vi "EDS test 02_2.vi"() -> ()   [LabVIEW 2020]
panel:
  out "max value":dbl
  in  "Ultrasonic 01":dbl
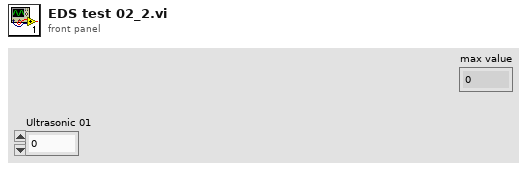
[diagram p1: front panel]
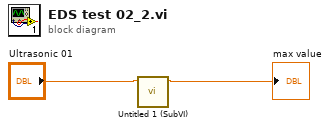
[diagram p0: block diagram]
diagram:
  n1 = call "Untitled 1 (SubVI).vi"("Ultrasonic 01"="Ultrasonic 01") -> ("Numeric"=→"max value":dbl)  [unwired: 10 in]
